vi "Acquire Session.vi"(8 "error in (no error)":errorcluster, 11 "session":T2) -> (0 "error out":errorcluster, 1 "abstract":T1, 2 "LIBSSH2_SESSION*":u64)   [LabVIEW 2017, in "libssh2.lvlib"]
uses:
  libssh2.lvlib
  Session Refnum.ctl
  libssh2_session_abstract.ctl
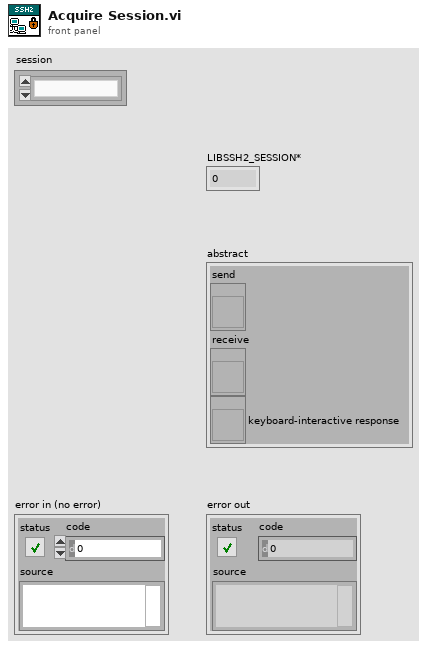
[diagram p1: front panel]
types:
  T1 = typedef "libssh2.lvlib/libssh2_session_abstract.ctl" = cluster{"send":refnum<vi>, "receive":refnum<vi>, "keyboard-interactive response":refnum<vi>}
  T2 = typedef "libssh2.lvlib/Session Refnum.ctl" = refnum<k1>
  T3 = typedef "Semaphore RefNum" = refnum<k1>
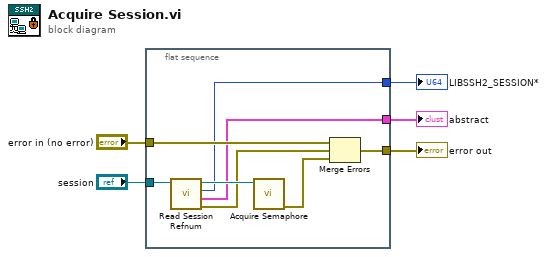
[diagram p0: block diagram]
diagram:
  n1 = flat-sequence {
    tunnel: [w10] -> w5
    tunnel: "error in (no error)" -> [w9]
    tunnel: "session" -> [w8]
    tunnel: [w7] -> w2
    tunnel: [w6] -> w1
    frame #0 {
      n2 = call "Read Session Refnum.vi"("session"=w8) -> ("error out"=w12:errorcluster, "abstract"=w6:T1, "LIBSSH2_SESSION*"=w7:u64, "semaphore"=w13:T3)  [unwired: 5 in, 2 out]
      n3 = call <vilib>:"Acquire Semaphore.vi"("semaphore"=w13) -> ("error out"=w11:errorcluster)  [unwired: 4 in, 2 out]
      n4 = Merge Errors(w9, w12, w11) -> (w10:errorcluster)
    }
  }
  "error out" <- w5
  "LIBSSH2_SESSION*" <- w2
  "abstract" <- w1
